vi "Transmit String Data.vi"() -> ()   [LabVIEW 2020, in "Test.lvlib"]
uses:
  Test.lvlib
  8b2a8d48-8f2b-4562-801b-642757049195.vi
  fea29164-ead3-404b-b2a8-9c1a4409b8f3.vi
  439305e5-3871-479c-9966-653eac169d2c.vi
  <vilib>/Utility/error.llb/Clear Errors.vi
  TCP Comms/Get Connected.vi
  <vilib>/Utility/error.llb/Error Cluster From Error Code.vi
  TCP Comms/Connection Ref.vi
  TCP Comms/Close TCP.vi
  TCP Comms/TinyTCP.lvlib
panel:
  out "Server Error":errorcluster
  out "Client Error":errorcluster
  out "Read String":string
  in  "To Send":string="Hello from sender!"
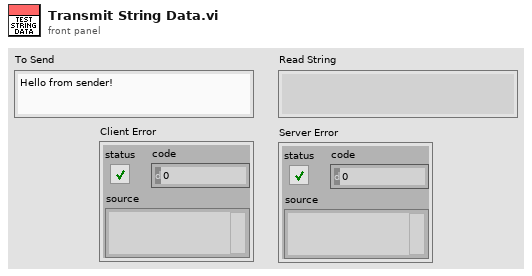
[diagram p1: front panel]
types:
  T1 = typedef "TinyTCP.lvlib/Instance.ctl" = refnum<data-value>
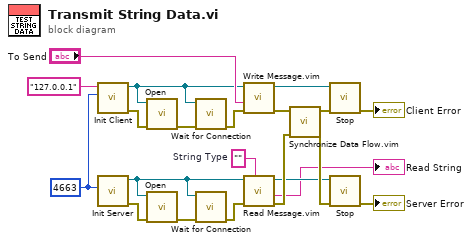
[diagram p0: block diagram]
diagram:
  w1 = ""  # String Type
  w18 = u16 4663 ("Port")
  n1 = call "Init Client.vi"("Port"=w18, "Host"="127.0.0.1") -> ("error out"=w17:errorcluster, "TinyTCP Client"=w4:T1)  [unwired: 8 in]
  n2 = call "Init Server.vi"("Port"=w18) -> ("error out"=w16:errorcluster, "TinyTCP Server"=w3:T1)  [unwired: 9 in]
  n3 = call "Open.vi"("error in (no error)"=w17, "TCP Comm"=w4) -> ("error out"=w6:errorcluster)  [unwired: 9 in]
  n4 = call "Open.vi"("error in (no error)"=w16, "TCP Comm"=w3) -> ("error out"=w7:errorcluster)  [unwired: 9 in]
  n5 = call "Wait for Connection.vi"("error in (no error)"=w6, "TinyTCP"=w4) -> ("error out"=w5:errorcluster)  [unwired: 9 in]
  n6 = call "Wait for Connection.vi"("error in (no error)"=w7, "TinyTCP"=w3) -> ("error out"=w2:errorcluster)  [unwired: 9 in]
  n7 = call "Write Message.vim"("error in (no error)"=w5, "Data"="To Send", "TCP Comm In"=w4) -> ("error out"=w14:errorcluster, "TCP Comm"=w12:T1)  [unwired: 6 in, 1 out]
  n8 = call "Read Message.vim"("Data Type (Raw Data)"=w1, "error in (no error)"=w2, "TCP Comm In"=w3) -> ("error out"=w20:errorcluster, "Data"=→"Read String":string, "TCP Comm"=w13:T1)  [unwired: 3 in, 3 out]
  n9 = call "Synchronize Data Flow.vim"("input 4"=w20, "input 1"=w14) -> ("output 4"=w21:errorcluster, "output 1"=w11:errorcluster)  [unwired: 2 in, 2 out]
  n10 = call "Stop.vi"("error in (no error)"=w11, "TCP Comm"=w12) -> ("error out"=→"Client Error":errorcluster)  [unwired: 9 in]
  n11 = call "Stop.vi"("error in (no error)"=w21, "TCP Comm"=w13) -> ("error out"=→"Server Error":errorcluster)  [unwired: 9 in]
